vi "example_plots.vi"() -> ()   [LabVIEW 2015]
panel:
  out "Plot 2":cluster{"X":dbl[], "Y":dbl[]}[](graph) caption="Absorption mHT profiles for H2-He (blue) and H2-Ar (orange)."
  out "Plot 1":cluster{"X":dbl[], "Y":dbl[]}[](graph) caption="Real (blue) and imaginary (orange) part for mHT output for H2-He"
  in  "alpha H2Ar":dbl=19.8186220035 caption="alpha (10)" format="%#_13g"
  in  "Ylm H2Ar":dbl caption="Ylm (0)" format="%#_13g"
  in  "Xlm H2Ar":dbl caption="Xlm (0)" format="%#_13g"
  in  "NuOptIm H2Ar":dbl=-0.0161 caption="NuOptIm (0)" format="%#_13g"
  in  "NuOptRe H2Ar":dbl=0.0721 caption="NuOptRe (0)" format="%#_13g"
  in  "Delta2 H2Ar":dbl=0.0178 caption="Delta2 (0)" format="%#_13g"
  in  "Gamma2 H2Ar":dbl=0.000374 caption="Gamma2 (0)" format="%#_13g"
  in  "Delta0 H2Ar":dbl=-0.0264 caption="Delta0 (0)" format="%#_13g"
  in  "Gamma0 H2Ar":dbl=0.0113 caption="Gamma0 (0)" format="%#_13g"
  in  "alpha H2He":dbl=1.98573285442 caption="alpha (10)" format="%#_13g"
  in  "Ylm H2He":dbl caption="Ylm (0)" format="%#_13g"
  in  "Xlm H2He":dbl caption="Xlm (0)" format="%#_13g"
  in  "NuOptIm H2He":dbl=-0.0175 caption="NuOptIm (0)" format="%#_13g"
  in  "NuOptRe H2He":dbl=0.038 caption="NuOptRe (0)" format="%#_13g"
  in  "Delta2 H2He":dbl=0.0124 caption="Delta2 (0)" format="%#_13g"
  in  "Gamma2 H2He":dbl=0.0054 caption="Gamma2 (0)" format="%#_13g"
  in  "Delta0 H2He":dbl=0.0305 caption="Delta0 (0)" format="%#_13g"
  in  "Gamma0 H2He":dbl=0.0117 caption="Gamma0 (0)" format="%#_13g"
  in  "GammaD":dbl=0.0351 caption="GammaD (0)" format="%#_13g"
  in  "nu0":dbl=112265.5949 caption="nu0 (0)" format="%#_13g"
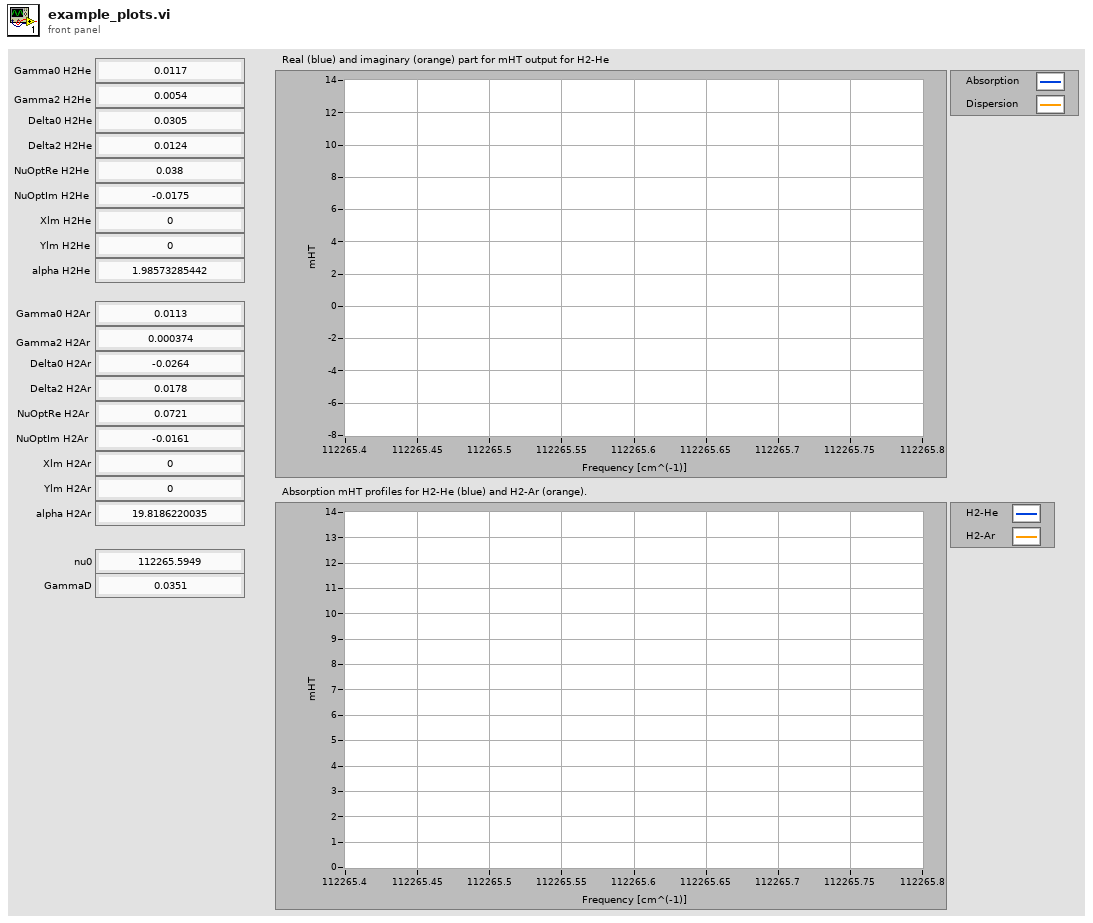
[diagram p1: front panel]
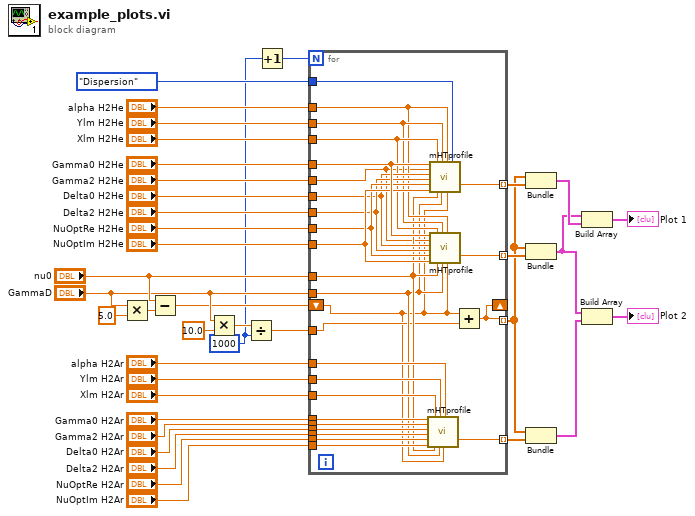
[diagram p0: block diagram]
diagram:
  w11 = 1000 ("y")
  n1 = Multiply(x="GammaD", y=5.0) -> (x*y=w19:dbl)
  n2 = Subtract(x="nu0", y=w19) -> (x-y=w12:dbl)
  n3 = Multiply(x="GammaD", y=10.0) -> (x*y=w14:dbl)
  n4 = Divide(x=w14, y=w11) -> (x/y=w13:dbl)
  n5 = Increment(x=w11) -> (x+1=w10:i32)
  n6 = for {
    N: w10 -> [_]
    tunnel: enum32{"Absorption", "Dispersion"}."Dispersion" ("disp") -> [w65]
    tunnel: "Gamma0 H2He" -> [w64]
    tunnel: "NuOptIm H2He" -> [w63]
    tunnel: "NuOptRe H2He" -> [w62]
    tunnel: "Delta2 H2He" -> [w61]
    tunnel: "Delta0 H2He" -> [w60]
    tunnel: "Xlm H2He" -> [w59]
    tunnel: "Ylm H2He" -> [w58]
    tunnel: "alpha H2He" -> [w57]
    tunnel: "Gamma0 H2Ar" -> [w56]
    tunnel: "Gamma2 H2Ar" -> [w55]
    tunnel: "Delta0 H2Ar" -> [w54]
    tunnel: "Delta2 H2Ar" -> [w53]
    tunnel: "NuOptRe H2Ar" -> [w52]
    tunnel: "NuOptIm H2Ar" -> [w51]
    tunnel: "Xlm H2Ar" -> [w50]
    tunnel: "Ylm H2Ar" -> [w49]
    tunnel: "alpha H2Ar" -> [w48]
    tunnel: "nu0" -> [w47]
    tunnel: "Gamma2 H2He" -> [w46]
    tunnel: "GammaD" -> [w45]
    tunnel: w13 -> [w44]
    shift-right: [w39] -> _
    shift-left: w12 -> [w43]
    tunnel: [w42] -> w7 mode=indexing
    tunnel: [w41] -> w8 mode=indexing
    tunnel: [w40] -> w9 mode=indexing
    tunnel: [w39] -> w6 mode=indexing
    n7 = call "mHTprofile.vi"("Gamma0"=w56, "Gamma2"=w55, "Delta0"=w54, "Delta2"=w53, "NuOptRe"=w52, "NuOptIm"=w51, "Xlm"=w50, "nu0"=w47, "Ylm"=w49, "GammaD"=w45, "alpha"=w48, "nu"=w43) -> ("mHT"=w42:dbl)  [unwired: 7 in]
    n8 = call "mHTprofile.vi"("Gamma0"=w64, "Gamma2"=w46, "Delta0"=w60, "Delta2"=w61, "NuOptRe"=w62, "NuOptIm"=w63, "Xlm"=w59, "nu0"=w47, "Ylm"=w58, "GammaD"=w45, "alpha"=w57, "nu"=w43, "disp"=w65) -> ("mHT"=w40:dbl)  [unwired: 6 in]
    n9 = call "mHTprofile.vi"("Gamma0"=w64, "Gamma2"=w46, "Delta0"=w60, "Delta2"=w61, "NuOptRe"=w62, "NuOptIm"=w63, "Xlm"=w59, "nu0"=w47, "Ylm"=w58, "GammaD"=w45, "alpha"=w57, "nu"=w43) -> ("mHT"=w41:dbl)  [unwired: 7 in]
    n10 = Add(x=w43, y=w44) -> (x+y=w39:dbl)
  }
  n11 = Bundle(w6, w9) -> (w5:cluster{dbl[], dbl[]})  [unwired: 1 in]
  n12 = Bundle(w6, w8) -> (w4:cluster{dbl[], dbl[]})  [unwired: 1 in]
  n13 = Bundle(w6, w7) -> (w3:cluster{dbl[], dbl[]})  [unwired: 1 in]
  n14 = Build Array(w4, w5) -> (→"Plot 1":cluster{dbl[], dbl[]}[])
  n15 = Build Array(w4, w3) -> (→"Plot 2":cluster{dbl[], dbl[]}[])
